vi "SlotNum Read.vi"(4 "error in (no error)":errorcluster, 6 "Container State":T3, 7 "Display State In":T1) -> (0 "error out":errorcluster, 2 "Value":i32, 3 "Display State Out":T1)   [LabVIEW 2020, in "PXISlot.xctl"]
uses:
  PXISlot.xctl
  <vilib>/_xctls/Container State.ctl
  State.ctl
  Connector Type.ctl
  <vilib>/_xctls/XControlSupport.lvlib
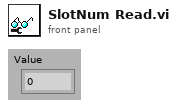
[diagram p1: front panel]
types:
  T1 = typedef "PXISlot.xctl/State.ctl" = cluster{"Connector Type":T2, "Hide unused":bool, "Type change?":bool, "Is dirty?":bool, "SlotNum":i32, "Trigger Visible":bool}
  T2 = typedef "Connector Type.ctl" = enum16{"None", "PXI-4461", "BNC-2110", "BNC-2090", "PXIe-4463", "PXIe-4464"}
  T3 = typedef "XControlSupport.lvlib/Container State.ctl" = cluster{"Indicator?":bool, "Run Mode?":bool, " Refnum":refnum<vi>}
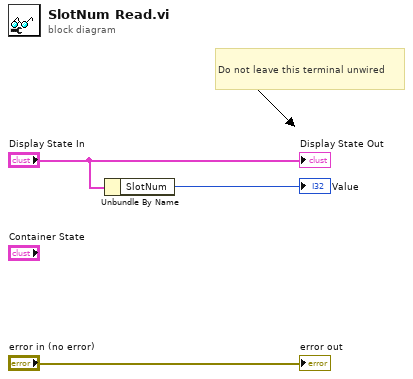
[diagram p0: block diagram]
diagram:
  # "Do not leave this terminal unwired"
  n1 = Unbundle By Name("Display State In") -> ("SlotNum"=→"Value":i32)
  "error out" <- "error in (no error)"
  "Display State Out" <- "Display State In"
